vi "FTP_Write.vi"(2 "Cmd":string, 3 "error in":errorcluster, 4 "data":string, 5 "connection ID in":refnum<k5>) -> (0 "error out":errorcluster, 1 "connection ID out":refnum<k5>)   [LabVIEW 2012]
uses:
  <userlib>/BotSpeak/Devices/EvalRIO/FTPCodes/FTPGlobals.vi
panel:
  in  "Task":T1(ring)
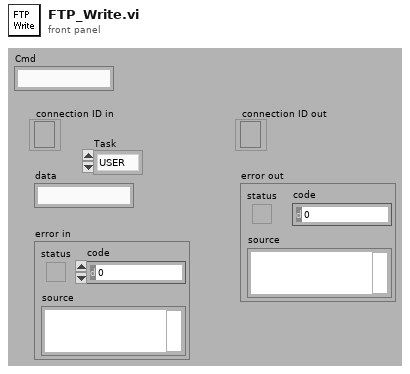
[diagram p1: front panel]
types:
  T1 = enum16{"USER", "PASS", "QUIT", "PASV", "STOR", "TYPE", "LIST", "CWD"}
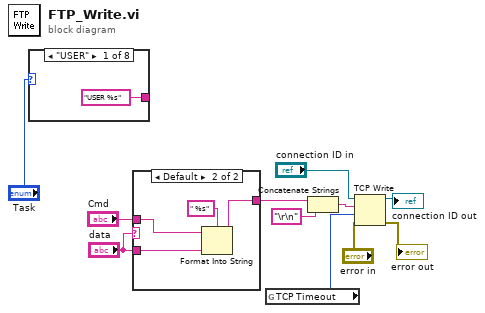
[diagram p0: block diagram]
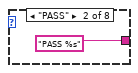
[diagram p3: hidden frame]
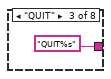
[diagram p4: hidden frame]
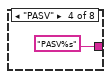
[diagram p5: hidden frame]
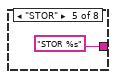
[diagram p6: hidden frame]
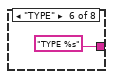
[diagram p7: hidden frame]
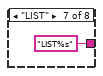
[diagram p8: hidden frame]
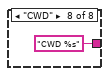
[diagram p9: hidden frame]
diagram:
  n1 = case shown="\"USER\"" "Task" {
    tunnel: ["USER %s" "PASS %s" "QUIT%s" "PASV%s" "STOR %s" "TYPE %s" "LIST%s" "CWD %s"] -> _
    frame "USER" {
    }
    frame "PASS" {
    }
    frame "QUIT" {
    }
    frame "PASV" {
    }
    frame "STOR" {
    }
    frame "TYPE" {
    }
    frame "LIST" {
    }
    frame "CWD" {
    }
  }
  n2 = case shown="Default" "data" {
    tunnel: "data" -> [_ w24]
    tunnel: [w20 w23] -> w4
    tunnel: "Cmd" -> [w20 w22]
    frame "" {
    }
    frame Default {
      n3 = Format Into String(format string=" %s", initial string=w22, w24) -> (resulting string=w23:string)  [unwired: 1 in, 1 out]
    }
  }
  n4 = global read "FTPGlobals.vi" "TCP Timeout"() -> (w1:i32)
  n5 = Concatenate Strings(w4, "\r\n" ("EOL (\\r\\n)")) -> (w7:string)
  n6 = TCP Write(connection ID="connection ID in", data in=w7, error in (no error)="error in", 9:w1) -> (connection ID out=→"connection ID out":refnum<k5>, error out=→"error out":errorcluster)  [unwired: 1 out]
